vi "_FPGA Check FPressure.vi"(4 "error in":errorcluster, 5 "DisableCheck (F)":bool, 6 "CheckNow (F)":bool) -> (0 "error out":errorcluster, 2 "PressureOK":bool)   [LabVIEW 2012]
uses:
  Type/_LCD Line2 Msg.ctl
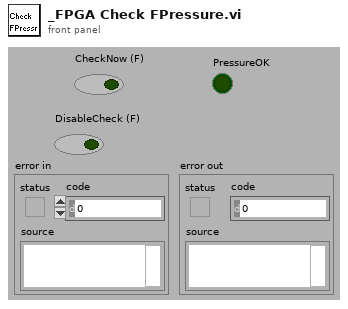
[diagram p1: front panel]
types:
  T1 = typedef "_LCD Line2 Msg.ctl" = u16
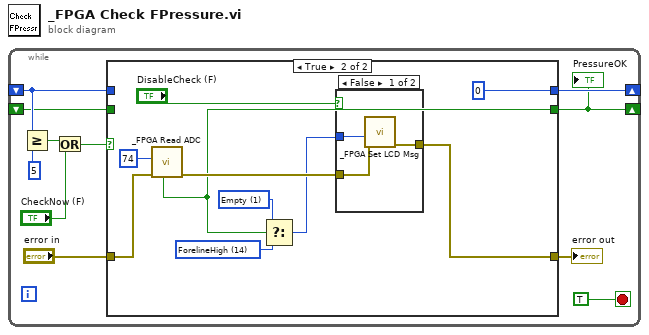
[diagram p0: block diagram]
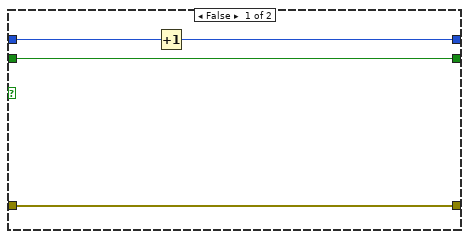
[diagram p2: hidden frame]
diagram:
  n1 = while {
    shift-right: [w10] -> _
    shift-left: _ -> [w5]
    shift-right: [w1] -> _
    shift-left: _ -> [w2]
    stop <- TRUE stop-if-true
    n2 = Greater Or Equal?(x=w5, y=5) -> (x >= y?=w8:bool)
    n3 = Or(x=w8, y="CheckNow (F)") -> (x .or. y?=w6:bool)
    n4 = case shown="True" w6 {
      tunnel: [w14 0] -> w10
      tunnel: w5 -> [w15 _]
      tunnel: [w13 w21] -> w3
      tunnel: "error in" -> [w13 w24]
      tunnel: [w12 w20] -> w1
      tunnel: w2 -> [w12 _]
      frame False {
        n5 = Increment(x=w15) -> (x+1=w14:i32)
      }
      frame True {
        w18 = T1 14 items=["Same", "Empty", "VacFail", "Cancel", "CheckGas", "EleFail", "Probe1Fail", "Probe2Fail", "HeaterFail", "DoorOpen", "CheckComm", "PressStart", "CheckSource", "VacWarn", "ForelineHigh"] ("Line2Msg (same)")
        w19 = T1 1 items=["Same", "Empty", "VacFail", "Cancel", "CheckGas", "EleFail", "Probe1Fail", "Probe2Fail", "HeaterFail", "DoorOpen", "CheckComm", "PressStart"] ("Line2Msg (same)")
        n6 = call "_FPGA Read ADC.vi"("error in"=w24, "ADC Channel (64)"=74) -> ("error out"=w22:errorcluster, "In Range?"=w20:bool)  [unwired: 1 in, 5 out]
        n7 = Select(t=w19, s=w20, f=w18) -> (s? t:f=w17:T1)
        n8 = case shown="False" "DisableCheck (F)" {
          tunnel: w22 -> [w28 w29]
          tunnel: [w27 w29] -> w21
          tunnel: w17 -> [w26 _]
          frame False {
            n9 = call "_FPGA Set LCD Msg.vi"("error in"=w28, "Line2Msg (same)"=w26) -> ("error out"=w27:errorcluster)  [unwired: 5 in, 2 out]
          }
          frame True {
          }
        }
      }
    }
    "error out" <- w3
    "PressureOK" <- w1
  }
